vi "meta_flush.vi"(8 "error in (no error)":errorcluster, 11 "meta file in":T1) -> (0 "error out":errorcluster, 3 "meta file out":T1)   [LabVIEW 2017, in "NI_ExcelFile.lvlib"]
uses:
  <vilib>/express/express shared/NI_ExcelFile/NI_ExcelFile.lvlib
  <vilib>/express/express shared/NI_ExcelFile/Ctrls/meta_file.ctl
  <vilib>/express/express shared/NI_ExcelFile/Ctrls/meta_Block.ctl
  <vilib>/express/express shared/NI_ExcelFile/Ctrls/meta_BlockType.ctl
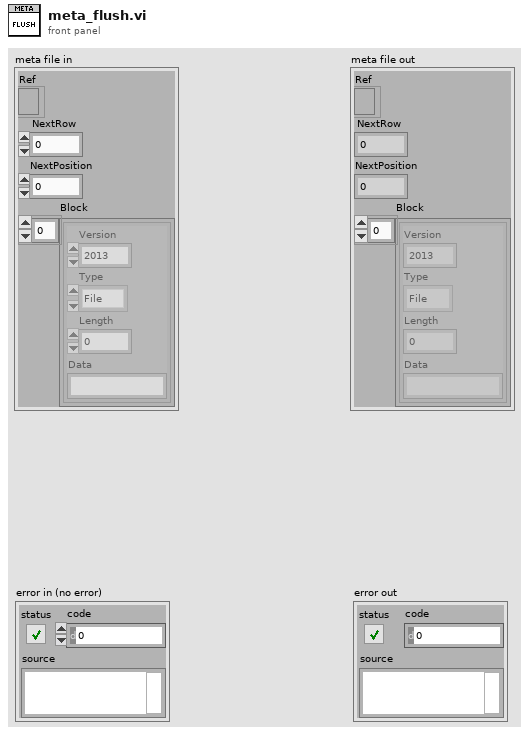
[diagram p1: front panel]
types:
  T1 = typedef "NI_ExcelFile.lvlib/meta_file.ctl" = cluster{"Ref":refnum<file>, "NextRow":i32, "NextPosition":i64, "Block":T2[]}
  T2 = typedef "NI_ExcelFile.lvlib/meta_Block.ctl" = cluster{"Version":u16, "Type":T3, "Length":i32, "Data":string}
  T3 = typedef "NI_ExcelFile.lvlib/meta_BlockType.ctl" = enum16{"NITag", "File", "Column"}
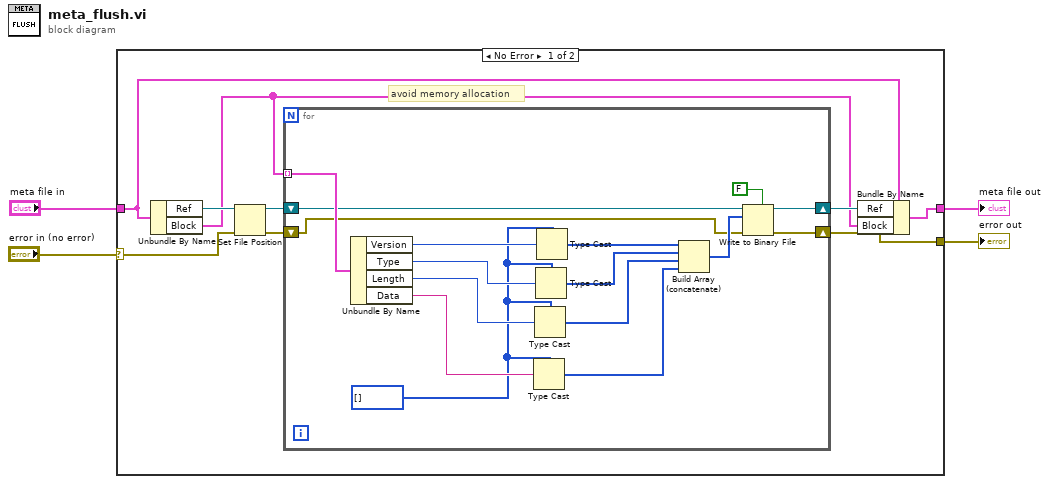
[diagram p0: block diagram]
diagram:
  n1 = case shown="No Error" "error in (no error)" {
    selector: "error in (no error)" -> [w6 w31]
    tunnel: "meta file in" -> [w10 w30]
    tunnel: [w13 w31] -> w2
    tunnel: [w12 w30] -> w1
    frame No Error {
      # "avoid memory allocation"
      n2 = Unbundle By Name(w10) -> ("Ref"=w9:refnum<file>, "Block"=w7:T2[])
      n3 = Set File Position(refnum=w9, error in=w6) -> (refnum out=w8:refnum<file>, error out=w5:errorcluster)  [unwired: 2 in]
      n4 = for {
        tunnel: w7 -> [w29] mode=indexing
        shift-right: [w15] -> w13
        shift-left: w5 -> [w16]
        shift-right: [w14] -> w11
        shift-left: w8 -> [w19]
        w20 = u8[] []
        n5 = Unbundle By Name(w29) -> ("Version"=w28:u16, "Type"=w27:T3, "Length"=w26:i32, "Data"=w25:string)
        n6 = Type Cast(type=w20, x=w25) -> (*(type *) &x=w21:u8[])
        n7 = Type Cast(type=w20, x=w26) -> (*(type *) &x=w22:u8[])
        n8 = Type Cast(type=w20, x=w27) -> (*(type *) &x=w23:u8[])
        n9 = Type Cast(type=w20, x=w28) -> (*(type *) &x=w24:u8[])
        n10 = Build Array (concatenate)(w24, w23, w22, w21) -> (w17:u8[])
        n11 = Write to Binary File(file (use dialog)=w19, data=w17, error in=w16, 5:FALSE ("prepend array or string size? (T)")) -> (refnum out=w14:refnum<file>, error out=w15:errorcluster)  [unwired: 2 in, 1 out]
      }
      n12 = Bundle By Name(cluster=w10, "Ref"=w11, "Block"=w7) -> (w12:T1)
    }
    frame Error {
    }
  }
  "meta file out" <- w1
  "error out" <- w2
